vi "Steriling Approx.vi"(10 "Large N":dbl) -> (2 "Approx.":dbl)   [LabVIEW 2017]
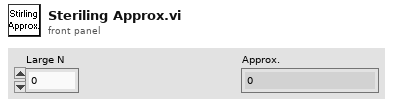
[diagram p1: front panel]
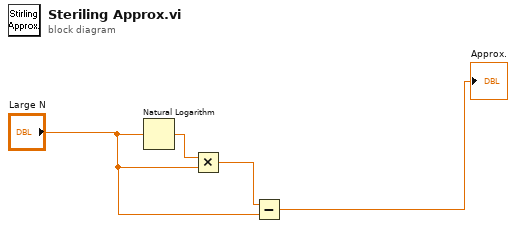
[diagram p0: block diagram]
diagram:
  n1 = Natural Logarithm(1:"Large N") -> (0:w4:dbl)
  n2 = Multiply(x=w4, y="Large N") -> (x*y=w3:dbl)
  n3 = Subtract(x=w3, y="Large N") -> (x-y=→"Approx.":dbl)
